vi "Get Configuration File from User.vi"(8 "error in":errorcluster) -> (0 "error out":errorcluster, 3 "Test Information":T1, 5 "selected path":path)   [LabVIEW 2015]
uses:
  Controls/Test Information.ctl
  Controls/Vacuum Test.ctl
  Controls/Test Timing.ctl
  Controls/Vaccum Thresholds.ctl
  Controls/Helium Test.ctl
  Controls/Helium Thresholds.ctl
  Controls/Startup Thresholds.ctl
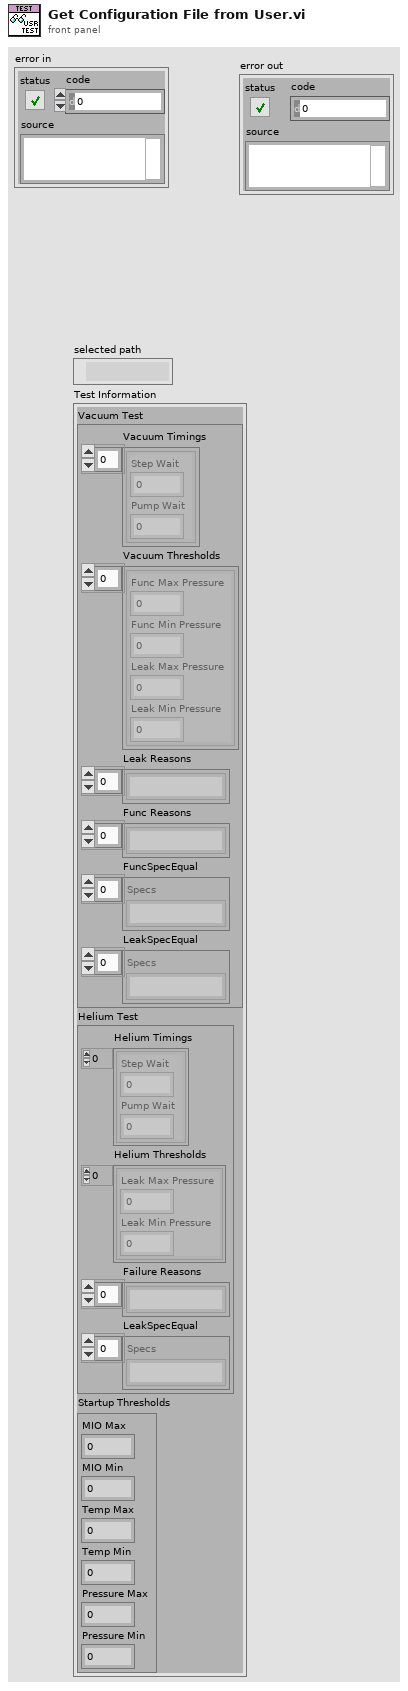
[diagram p1: front panel]
types:
  T1 = typedef "Test Information.ctl" = cluster{"Vacuum Test":T2, "Helium Test":T5, "Startup Thresholds":T7}
  T2 = typedef "Vacuum Test.ctl" = cluster{"Vacuum Timings":T3[], "Vacuum Thresholds":T4[], "Leak Reasons":string[], "Func Reasons":string[], "FuncSpecEqual":string[], "LeakSpecEqual":string[]}
  T3 = typedef "Test Timing.ctl" = cluster{"Step Wait":dbl, "Pump Wait":dbl}
  T4 = typedef "Vaccum Thresholds.ctl" = cluster{"Func Max Pressure":dbl, "Func Min Pressure":dbl, "Leak Max Pressure":dbl, "Leak Min Pressure":dbl}
  T5 = typedef "Helium Test.ctl" = cluster{"Helium Timings":T3[], "Helium Thresholds":T6[], "Failure Reasons":string[], "LeakSpecEqual":string[]}
  T6 = typedef "Helium Thresholds.ctl" = cluster{"Leak Max Pressure":dbl, "Leak Min Pressure":dbl}
  T7 = typedef "Startup Thresholds.ctl" = cluster{"MIO Max":dbl, "MIO Min":dbl, "Temp Max":dbl, "Temp Min":dbl, "Pressure Max":dbl, "Pressure Min":dbl}
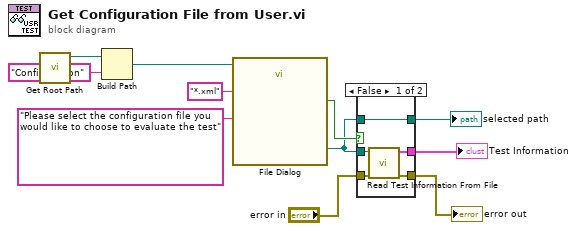
[diagram p0: block diagram]
diagram:
  n1 = call "Get Root Path.vi"() -> ("Root Path"=w10:path)  [unwired: 11 in]
  n2 = Build Path(base path=w10, name or relative path="Configuration") -> (appended path=w9:path)
  n3 = call "File Dialog"("start path"=w9, "prompt"="Please select the configuration file you would like to choose to evaluate the test", "pattern (all files)"="*.xml") -> ("selected path"=w3:path, "cancelled"=w5:bool)  [unwired: 9 in, 2 out]
  n4 = case shown="False" w5 {
    tunnel: "error in" -> [w16 w17]
    tunnel: w3 -> [w15 _]
    tunnel: [w14 _] -> w1
    tunnel: [w13 w17] -> w6
    tunnel: [w12 _] -> w2
    tunnel: w3 -> [w12 _]
    frame False {
      n5 = call "Read Test Information From File.vi"("error in"=w16, "file (use dialog)"=w15) -> ("error out"=w13:errorcluster, "Test Information"=w14:T1)  [unwired: 8 in]
    }
    frame True {
    }
  }
  "error out" <- w6
  "selected path" <- w2
  "Test Information" <- w1
